vi "HXG2_Data Process.vi"(8 "error in":errorcluster, 9 "Analog DATA In":T3, 10 "BoolSelection In":T2, 11 "Calculated Values":T1) -> (0 "error out":errorcluster, 3 "Calculated Values":T1)   [LabVIEW 2012]
doc: "This VI calculates all averages, heat loads, RH, etc..."
uses:
  Controls/HXG2_AnalogIn.ctl
  Controls/HXG2_BooleanSelections.ctl
  Controls/HXG2_Calculated.ctl
  <vilib>/addons/control/pid/pid.llb/PID Control Input Filter (DBL).vi
  <vilib>/addons/control/pid/NI_PID_pid.lvlib
panel:
  in  "reinitialize?\nMdot Filter (F)":bool
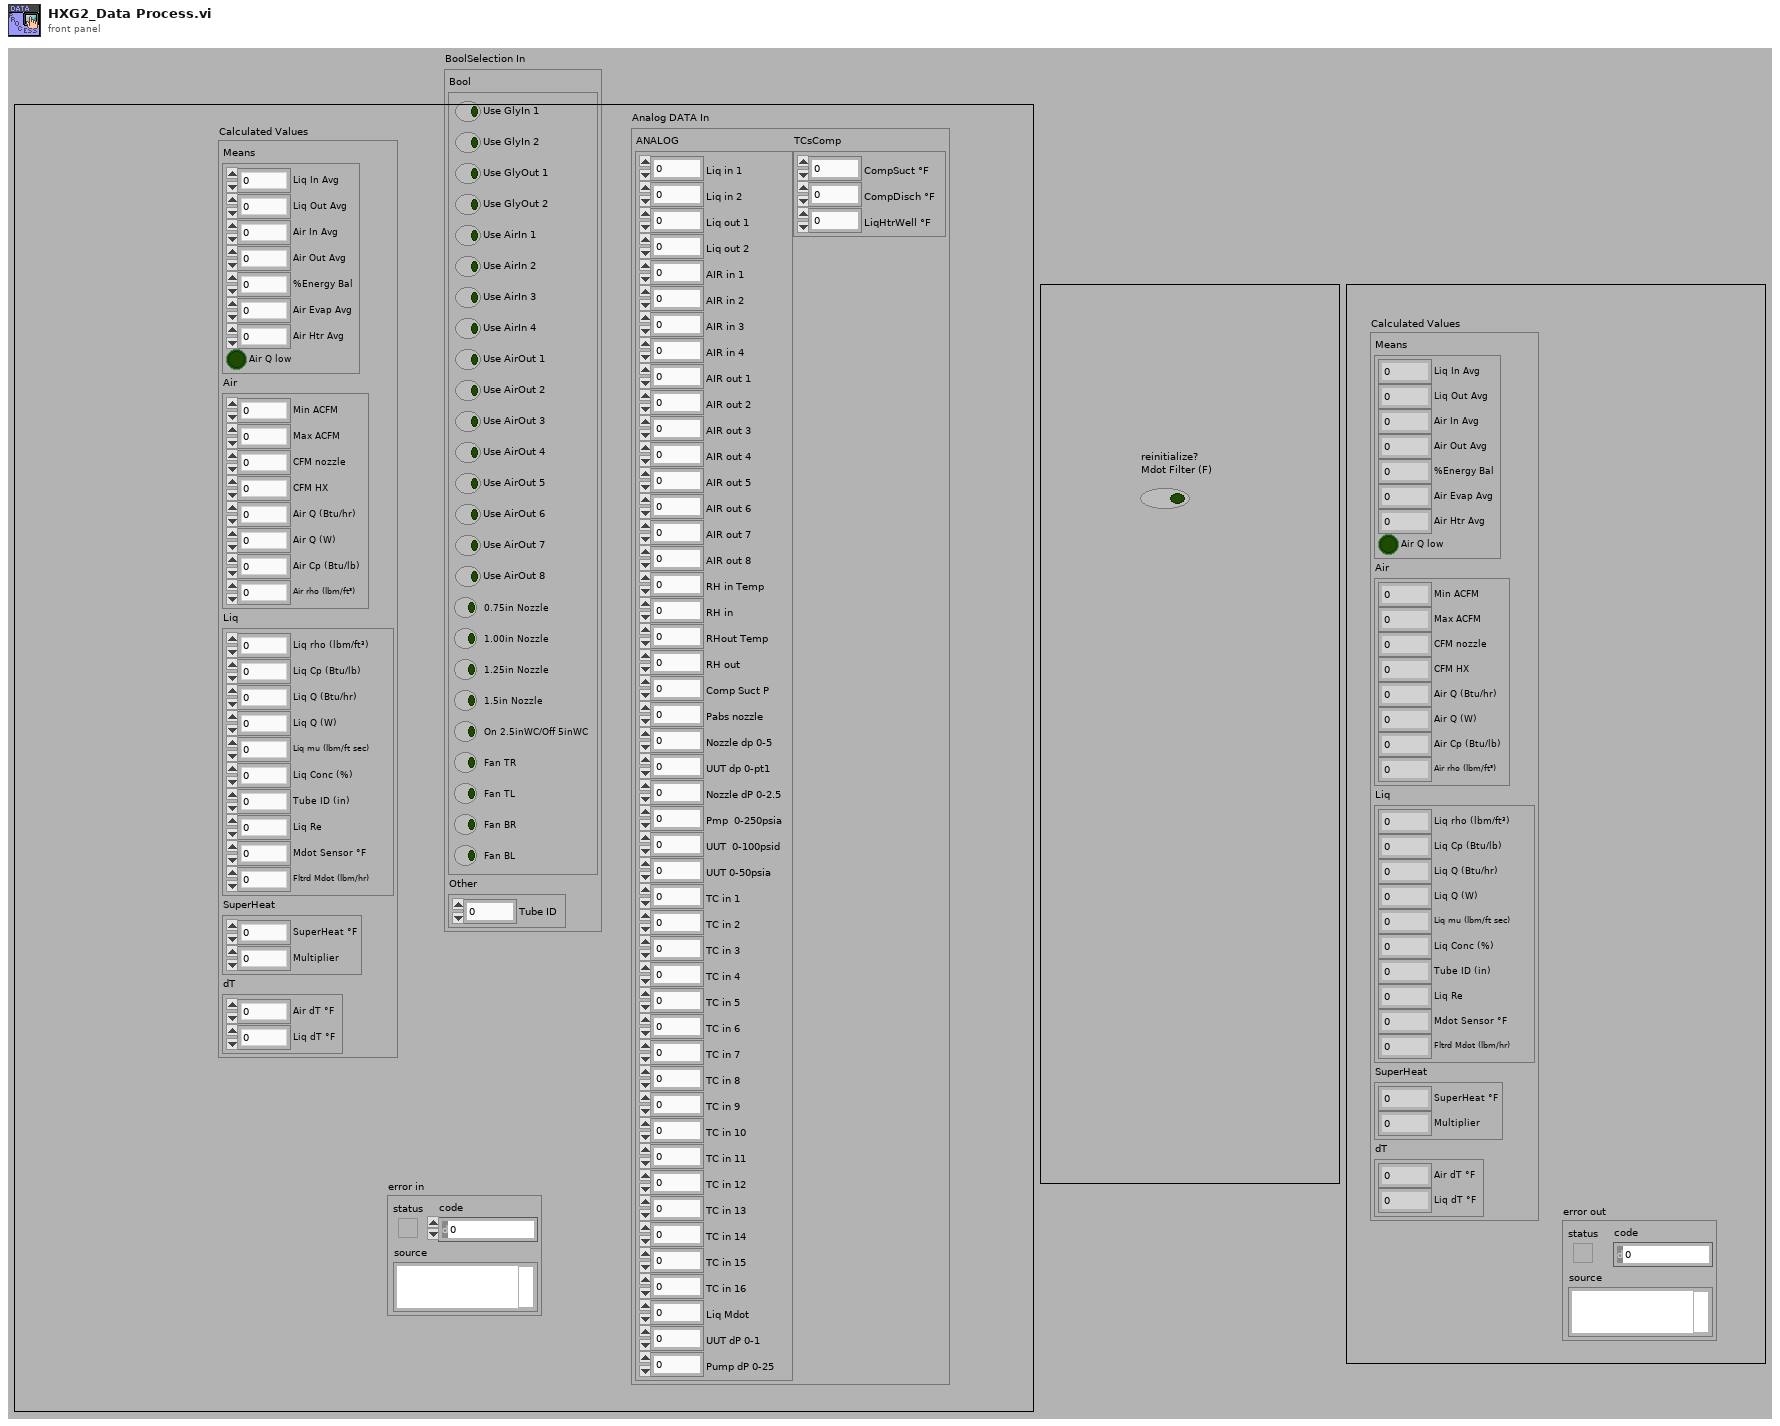
[diagram p1: front panel]
types:
  T1 = typedef "HXG2_Calculated.ctl" = cluster{"Means":cluster{"Liq In Avg":dbl, "Liq Out Avg":dbl, "Air In Avg":dbl, "Air Out Avg":dbl, "%Energy Bal":dbl, "Air Evap Avg":dbl, "Air Htr Avg":dbl, "Air Q low":bool}, "Air":cluster{"Min ACFM":dbl, "Max ACFM":dbl, "CFM nozzle":dbl, "CFM HX":dbl, "Air Q (Btu/hr)":dbl, "Air Q (W)":dbl, "Air Cp (Btu/lb)":dbl, "Air rho (lbm/ft³)":dbl}, "Liq":cluster{"Liq rho (lbm/ft³)":dbl, "Liq Cp (Btu/lb)":dbl, "Liq Q (Btu/hr)":dbl, "Liq Q (W)":dbl, "Liq mu (lbm/ft sec)":dbl, "Liq Conc (%)":dbl, "Tube ID (in)":dbl, "Liq Re":dbl, "Mdot Sensor °F":dbl, "Fltrd Mdot (lbm/hr)":dbl}, "SuperHeat":cluster{"SuperHeat °F":dbl, "Multiplier":dbl}, "dT":cluster{"Air dT °F":dbl, "Liq dT °F":dbl}}
  T2 = typedef "HXG2_BooleanSelections.ctl" = cluster{"Bool":cluster{"Use GlyIn 1":bool, "Use GlyIn 2":bool, "Use GlyOut 1":bool, "Use GlyOut 2":bool, "Use AirIn 1":bool, "Use AirIn 2":bool, "Use AirIn 3":bool, "Use AirIn 4":bool, "Use AirOut 1":bool, "Use AirOut 2":bool, "Use AirOut 3":bool, "Use AirOut 4":bool, "Use AirOut 5":bool, "Use AirOut 6":bool, "Use AirOut 7":bool, "Use AirOut 8":bool, "0.75in Nozzle":bool, "1.00in Nozzle":bool, "1.25in Nozzle":bool, "1.5in Nozzle":bool, "On 2.5inWC/Off 5inWC":bool, "Fan TR":bool, "Fan TL":bool, "Fan BR":bool, "Fan BL":bool}, "Other":cluster{"Tube ID":dbl}}
  T3 = typedef "HXG2_AnalogIn.ctl" = cluster{"ANALOG":cluster{"Liq in 1":dbl, "Liq in 2":dbl, "Liq out 1":dbl, "Liq out 2":dbl, "AIR in 1":dbl, "AIR in 2":dbl, "AIR in 3":dbl, "AIR in 4":dbl, "AIR out 1":dbl, "AIR out 2":dbl, "AIR out 3":dbl, "AIR out 4":dbl, "AIR out 5":dbl, "AIR out 6":dbl, "AIR out 7":dbl, "AIR out 8":dbl, "RH in Temp":dbl, "RH in":dbl, "RHout Temp":dbl, "RH out":dbl, "Comp Suct P":dbl, "Pabs nozzle":dbl, "Nozzle dp 0-5":dbl, "UUT dp 0-pt1":dbl, "Nozzle dP 0-2.5":dbl, "Pmp  0-250psia":dbl, "UUT  0-100psid":dbl, "UUT 0-50psia":dbl, "TC in 1":dbl, "TC in 2":dbl, "TC in 3":dbl, "TC in 4":dbl, "TC in 5":dbl, "TC in 6":dbl, "TC in 7":dbl, "TC in 8":dbl, "TC in 9":dbl, "TC in 10":dbl, "TC in 11":dbl, "TC in 12":dbl, "TC in 13":dbl, "TC in 14":dbl, "TC in 15":dbl, "TC in 16":dbl, "Liq Mdot":dbl, "UUT dP 0-1":dbl, "Pump dP 0-25":dbl}, "TCsComp":cluster{"CompSuct °F  ":dbl, "CompDisch °F":dbl, "LiqHtrWell °F":dbl}}
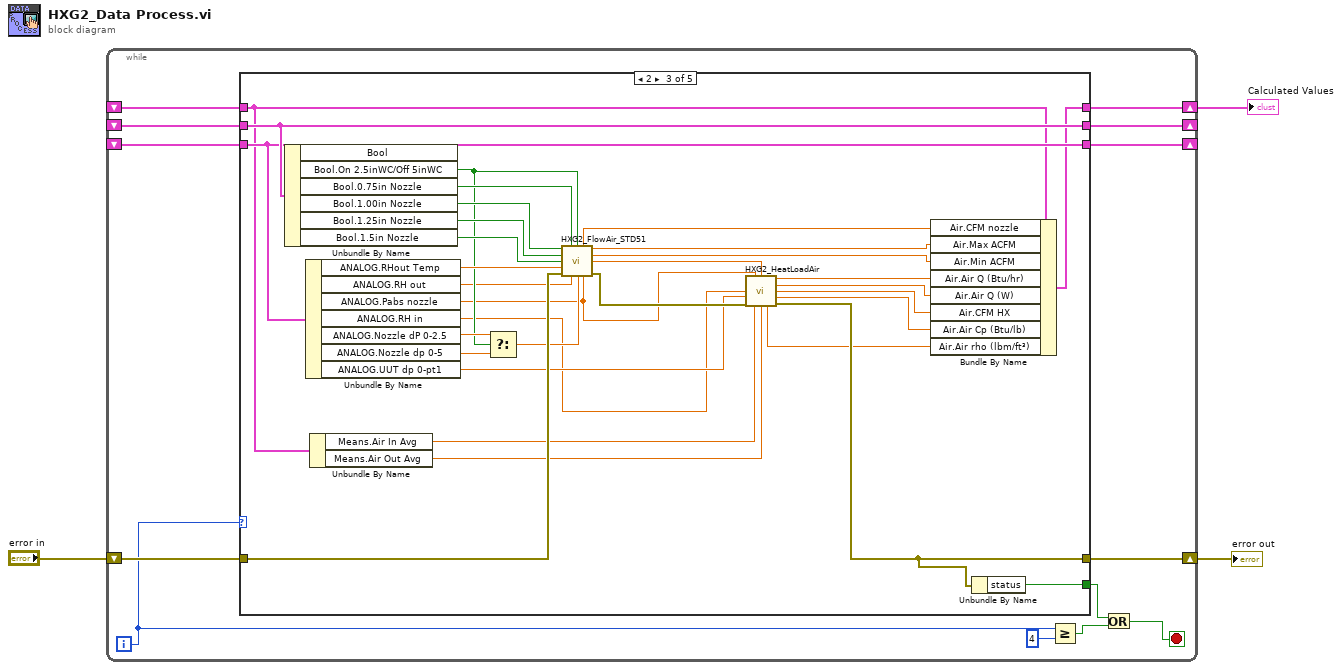
[diagram p0: block diagram]
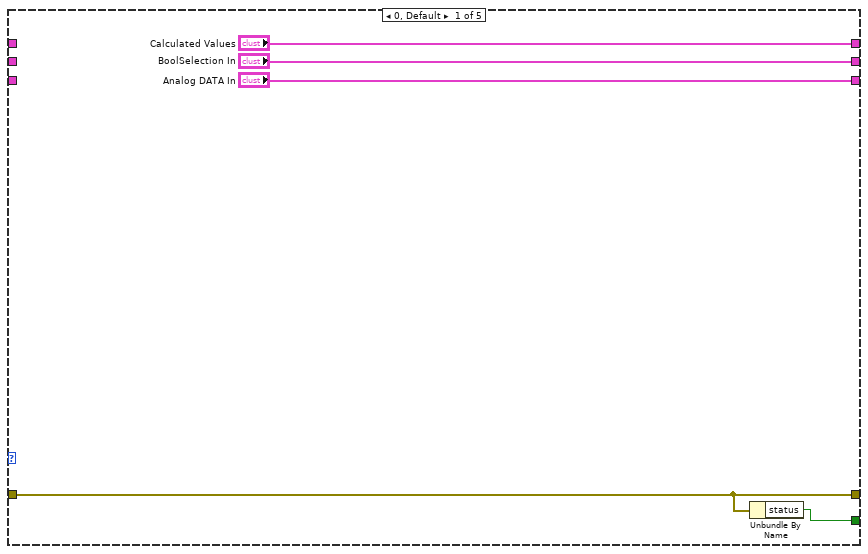
[diagram p2: hidden frame]
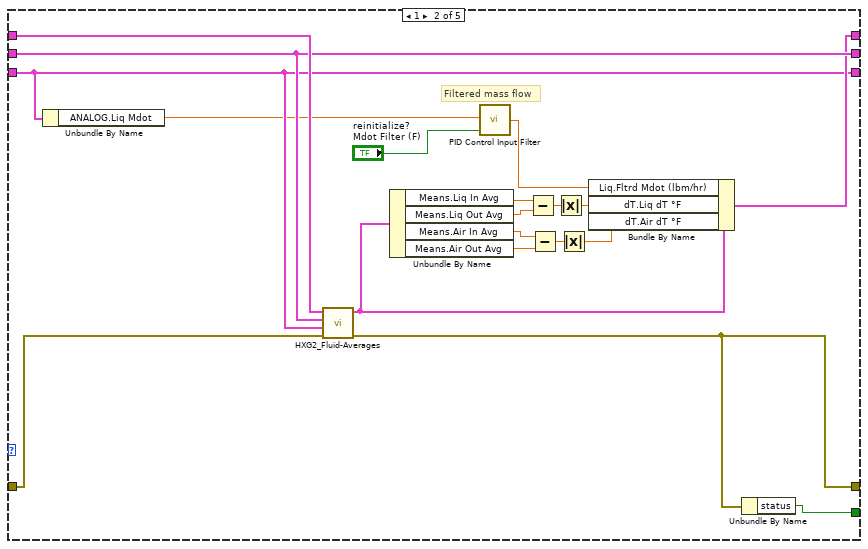
[diagram p3: hidden frame]
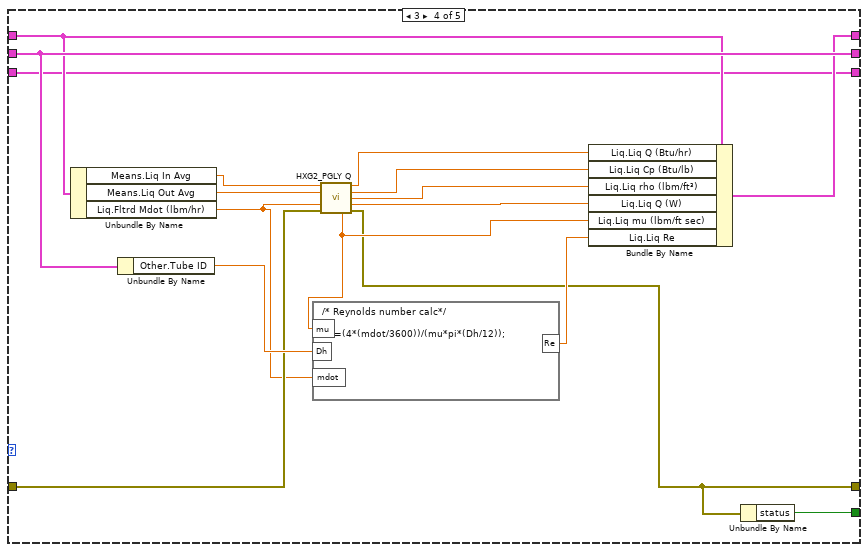
[diagram p4: hidden frame]
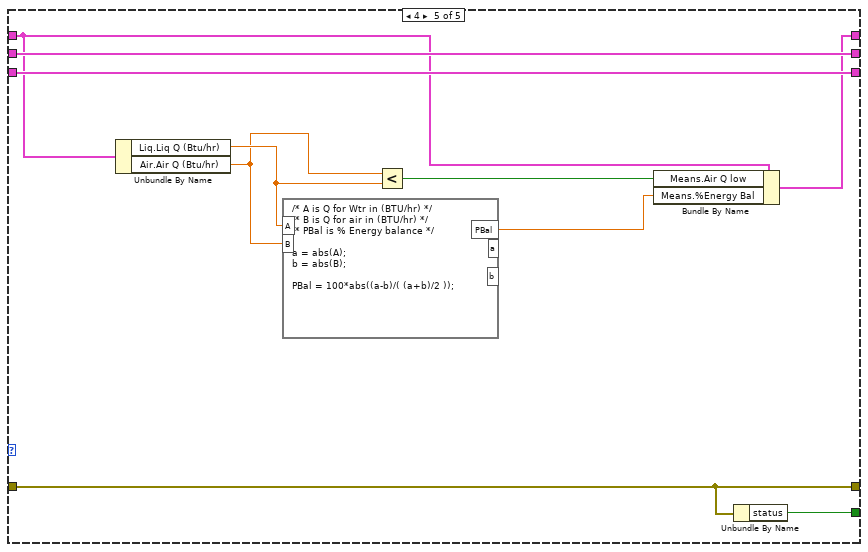
[diagram p5: hidden frame]
diagram:
  n1 = while {
    shift-right: [w16] -> w1
    shift-left: _ -> [w14]
    shift-right: [w15] -> _
    shift-left: _ -> [w13]
    shift-right: [w12] -> _
    shift-left: _ -> [w11]
    shift-right: [w9] -> w3
    shift-left: "error in" -> [w10]
    i -> [w5]
    stop <- w6 stop-if-true
    n2 = case shown="2" w5 {
      tunnel: ["Calculated Values" w26 w63 w81 w92] -> w16
      tunnel: ["BoolSelection In" w38 w67 w83 w99] -> w15
      tunnel: w14 -> [_ w39 w64 w82 w93]
      tunnel: w13 -> [_ w38 w67 w83 w99]
      tunnel: ["Analog DATA In" w25 w66 w75 w98] -> w12
      tunnel: w11 -> [_ w25 w66 w75 w98]
      tunnel: w10 -> [w18 w40 w65 w80 w91]
      tunnel: [w18 w37 w56 w78 w91] -> w9
      tunnel: [w17 w36 w55 w77 w90] -> w8
      frame 0, Default {
        n3 = Unbundle By Name(w18) -> ("status"=w17:bool)
      }
      frame 1 {
        # "Filtered mass flow"
        n4 = Unbundle By Name(w25) -> ("ANALOG.Liq Mdot"=w24:dbl)
        n5 = call "HXG2_Fluid-Averages.vi"("error in (no error)"=w40, "Analog DATA In"=w25, "BoolSelection In"=w38, "CalcValues"=w39) -> ("error out"=w37:errorcluster, "Calculated Values"=w35:T1)  [unwired: 6 in]
        n6 = Unbundle By Name(w35) -> ("Means.Liq In Avg"=w34:dbl, "Means.Liq Out Avg"=w33:dbl, "Means.Air In Avg"=w31:dbl, "Means.Air Out Avg"=w32:dbl)
        n7 = call-poly <vilib>:"PID Control Input Filter.vi"("reinitialize? (F)"="reinitialize?\nMdot Filter (F)", "input"=w24) -> ("output"=w23:dbl)  [unwired: 3 in]
        n8 = Subtract(x=w34, y=w33) -> (x-y=w30:dbl)
        n9 = Subtract(x=w31, y=w32) -> (x-y=w29:dbl)
        n10 = Absolute Value(x=w30) -> (abs(x)=w28:dbl)
        n11 = Absolute Value(x=w29) -> (abs(x)=w27:dbl)
        n12 = Bundle By Name(cluster=w35, "Liq.Fltrd Mdot (lbm/hr)"=w23, "dT.Liq dT °F"=w28, "dT.Air dT °F"=w27) -> (w26:T1)
        n13 = Unbundle By Name(w37) -> ("status"=w36:bool)
      }
      frame 2 {
        n14 = Unbundle By Name(w67) -> ("Bool.On 2.5inWC/Off 5inWC"=w51:bool, "Bool.0.75in Nozzle"=w69:bool, "Bool.1.00in Nozzle"=w70:bool, "Bool.1.25in Nozzle"=w71:bool, "Bool.1.5in Nozzle"=w72:bool)  [unwired: 1 out]
        n15 = Unbundle By Name(w66) -> ("ANALOG.RHout Temp"=w68:dbl, "ANALOG.RH out"=w48:dbl, "ANALOG.Pabs nozzle"=w49:dbl, "ANALOG.RH in"=w41:dbl, "ANALOG.Nozzle dP 0-2.5"=w54:dbl, "ANALOG.Nozzle dp 0-5"=w53:dbl, "ANALOG.UUT dp 0-pt1"=w47:dbl)
        n16 = Unbundle By Name(w64) -> ("Means.Air In Avg"=w58:dbl, "Means.Air Out Avg"=w59:dbl)
        n17 = Select(t=w54, s=w51, f=w53) -> (s? t:f=w52:dbl)
        n18 = call "HXG2_FlowAir_STD51.vi"("1\" Nozzle"=w70, "0.75\" Nozzle"=w69, "2.5inWC Sensor?"=w51, "1.25\" Nozzle"=w71, "1.5\" Nozzle"=w72, "Nozzle in Td °F"=w68, "error in (no error)"=w65, "Nozzle in %RH"=w48, "Nozzle DP inWC"=w52, "Pbarometric psi"=w49) -> ("CFM Nozzle"=w50:dbl, "MaxSCFM"=w62:dbl, "MinSCFM"=w61:dbl, "Mdot (lbm/hr)"=w57:dbl, "error out"=w60:errorcluster)  [unwired: 1 out]
        n19 = call "HXG2_HeatLoadAir.vi"("Pbaro (psia)"=w49, "Mdot Air (lbm/hr)"=w57, "%RH UUT"=w41, "dP UUT (inWC)"=w47, "error in (no error)"=w60, "Air In Avg (°F)"=w58, "Air Out Avg (°F)"=w59) -> ("Q air (BTU/hr)"=w46:dbl, "Qair (W)"=w45:dbl, "CFM HX"=w44:dbl, "Moist Air Cp (BTU/lb)"=w43:dbl, "Moist Air Density (lbm/ft³)"=w42:dbl, "error out"=w56:errorcluster)  [unwired: 3 in]
        n20 = Bundle By Name(cluster=w64, "Air.CFM nozzle"=w50, "Air.Max ACFM"=w62, "Air.Min ACFM"=w61, "Air.Air Q (Btu/hr)"=w46, "Air.Air Q (W)"=w45, "Air.CFM HX"=w44, "Air.Air Cp (Btu/lb)"=w43, "Air.Air rho (lbm/ft³)"=w42) -> (w63:T1)
        n21 = Unbundle By Name(w56) -> ("status"=w55:bool)
      }
      frame 3 {
        n22 = Unbundle By Name(w82) -> ("Means.Liq In Avg"=w74:dbl, "Means.Liq Out Avg"=w73:dbl, "Liq.Fltrd Mdot (lbm/hr)"=w76:dbl)
        n23 = Unbundle By Name(w83) -> ("Other.Tube ID"=w87:dbl)
        n24 = call "HXG2_PGLY Q.vi"("Liq In Avg. (°F)"=w74, "Liq Out Avg. (°F)"=w73, "Liq Flow (lbm/hr)"=w76, "error in (no error)"=w80) -> ("Q Wtr (BTU/hr)"=w85:dbl, "Cp (btu/lb)"=w84:dbl, "Density (lbm/ft³)"=w89:dbl, "Q Wtr (W)"=w88:dbl, "mu (lbm/ft*s)"=w86:dbl, "error out"=w78:errorcluster)  [unwired: 6 in]
        n25 = formula code="/* Reynolds number calc*/\n\nRe=(4*(mdot/3600))/(mu*pi*(Dh/12));"("Dh"=w87, "mu"=w86, "mdot"=w76) -> ("Re"=w79:dbl)
        n26 = Bundle By Name(cluster=w82, "Liq.Liq Q (Btu/hr)"=w85, "Liq.Liq Cp (Btu/lb)"=w84, "Liq.Liq rho (lbm/ft³)"=w89, "Liq.Liq Q (W)"=w88, "Liq.Liq mu (lbm/ft sec)"=w86, "Liq.Liq Re"=w79) -> (w81:T1)
        n27 = Unbundle By Name(w78) -> ("status"=w77:bool)
      }
      frame 4 {
        n28 = Unbundle By Name(w93) -> ("Liq.Liq Q (Btu/hr)"=w96:dbl, "Air.Air Q (Btu/hr)"=w95:dbl)
        n29 = formula code="/* A is Q for Wtr in (BTU/hr) */\n/* B is Q for air in (BTU/hr) */\n/* PBal is % Energy balance */\n\na = abs(A);\nb = abs(B);\n\nPBal = 100*abs((a-b)/( (a+b)/2 ));"("A"=w96, "B"=w95) -> ("PBal"=w94:dbl)  [unwired: 2 out]
        n30 = Less?(x=w95, y=w96) -> (x < y?=w97:bool)
        n31 = Bundle By Name(cluster=w93, "Means.Air Q low"=w97, "Means.%Energy Bal"=w94) -> (w92:T1)
        n32 = Unbundle By Name(w91) -> ("status"=w90:bool)
      }
    }
    n33 = Greater Or Equal?(x=w5, y=4) -> (x >= y?=w7:bool)
    n34 = Or(x=w8, y=w7) -> (x .or. y?=w6:bool)
  }
  "error out" <- w3
  "Calculated Values" <- w1
